vi "Get Current Lock State.vi"(8 "error in":errorcluster, 11 "EL Control Load CFG in":refnum<class "EL Control Load CFG.lvclass">) -> (0 "error out":errorcluster, 2 "Lock State":enum16{"NONE", "LOCAL", "REMOTE"}(ring), 3 "EL Control Load CFG out":refnum<class "EL Control Load CFG.lvclass">)   [LabVIEW 2023, in "EL Control Load CFG.lvclass"]
uses:
  EL Control Load CFG.lvclass
  EL Control Load CFG.lvclass/EL Control Load CFG.ctl
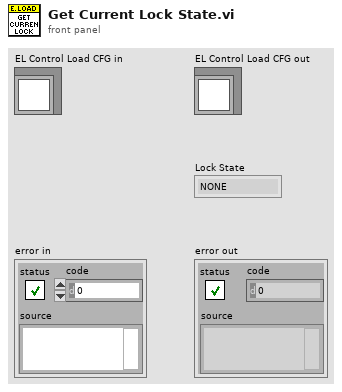
[diagram p1: front panel]
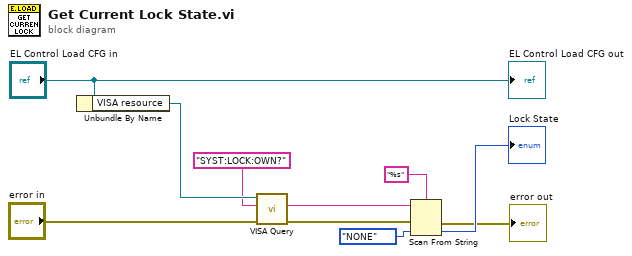
[diagram p0: block diagram]
diagram:
  n1 = Unbundle By Name("EL Control Load CFG in") -> ("VISA resource"=w9:refnum<visa-resource-name>)
  n2 = call "VISA Query.vi"("error in (no error)"="error in", "write buffer"="SYST:LOCK:OWN?", "VISA Refnum in"=w9) -> ("error out"=w2:errorcluster, "read buffer"=w7:string)  [unwired: 6 in, 1 out]
  n3 = Scan From String(format string="%s", input string=w7, error in=w2, default 1=enum16{"NONE", "LOCAL", "REMOTE"}."NONE" ("Enum")) -> (error out=→"error out":errorcluster, output 1=→"Lock State":enum16{"NONE", "LOCAL", "REMOTE"})  [unwired: 1 in, 2 out]
  "EL Control Load CFG out" <- "EL Control Load CFG in"
